vi "Check for items.vi"(11 "BYU ID # In":string) -> (3 "No Items":bool)   [LabVIEW 2019]
uses:
  <vilib>/addons/database/Auxilliary.llb/DB Tools Cursor Type.ctl
  <vilib>/addons/database/Connection.llb/DB Tools Open Connec (String).vi
  <vilib>/addons/database/Connection.llb/Conn Execute.vi
  <vilib>/addons/database/Recordset.llb/Rec Fetch Recordset Data (R).vi
  <vilib>/addons/database/Recordset.llb/Rec Destroy - Connection.vi
  <vilib>/addons/database/_DB Variant To Data/Database Variant To Data.xnode
  <vilib>/addons/database/NI_Database_API.lvlib
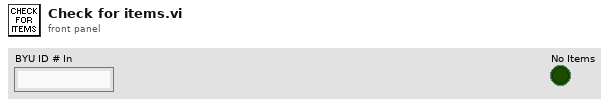
[diagram p1: front panel]
types:
  T1 = typedef "NI_Database_API.lvlib/DB Tools Cursor Type.ctl" = enum16{"forward-only", "keyset", "dynamic", "static"}
  T2 = typedef "NI_Database_API.lvlib/Conn ObjectReference.ctl" = refnum<k1>
  T3 = typedef "NI_Database_API.lvlib/Rec ObjectReference.ctl" = refnum<k1>
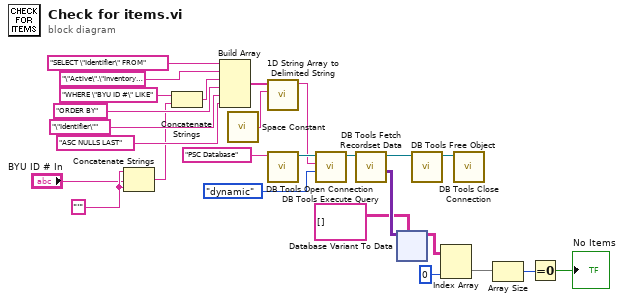
[diagram p0: block diagram]
diagram:
  w9 = "'"
  n1 = Concatenate Strings(w9, "BYU ID # In", w9) -> (w10:string)
  n2 = Concatenate Strings("WHERE \"BYU ID #\" LIKE", w10) -> (w22:string)
  n3 = Build Array("SELECT \"Identifier\" FROM", "\"Active\".\"Inventory\"", w22, "ORDER BY", "\"Identifier\"", "ASC NULLS LAST") -> (w20:string[])
  n4 = call <vilib>:"Space Constant.vi"() -> ("String"=w19:string)
  n5 = call <vilib>:"1D String Array to Delimited String.vi"("delimiter"=w19, "string array"=w20) -> ("delimited string"=w18:string)  [unwired: 9 in]
  n6 = call-poly <vilib>:"DB Tools Open Connection.vi"("connection information"="PSC Database") -> ("connection reference"=w26:T2)  [unwired: 7 in, 1 out]
  n7 = call-poly <vilib>:"DB Tools Execute Query.vi"("cursor type"=DB_Tools_Cursor_Type."dynamic", "SQL query"=w18, "connection reference"=w26) -> ("recordset reference"=w16:T3)  [unwired: 5 in, 1 out]
  n8 = call-poly <vilib>:"DB Tools Fetch Recordset Data.vi"("recordset reference"=w16) -> ("recordset data"=w7:variant[][], "recordset reference out"=w15:T3)  [unwired: 4 in, 1 out]
  n9 = xnode "Database Variant To Data"("database variant"=w7, "type"=string[][] []) -> ("data"=w5:string[][])  [unwired: 1 in, 1 out]
  n10 = call-poly <vilib>:"DB Tools Free Object.vi"("recordset reference"=w15) -> ("connection reference"=w14:T2)  [unwired: 9 in, 1 out]
  n11 = Index Array(array=w5, index (col)=0 ("disabled index (col)")) -> (element=w3:string[])  [unwired: 1 in]
  n12 = call <vilib>:"DB Tools Close Connection.vi"("connection reference"=w14) -> ()  [unwired: 6 in, 1 out]
  n13 = Array Size(array=w3) -> (size(s)=w2:i32)
  n14 = Equal To 0?(x=w2) -> (x = 0?=→"No Items":bool)
